vi "LVPortInitMatlab.vi"(0 "Working directory or VI Path":path, 1 "LVPort Code Lib Path (If empty auto find)":path, 5 "Code file name":string, 7 "Include path":path, 9 "Include Paths":path[](array[path]), 11 "error in":errorcluster, 12 "Autofind CodeFile if not provided":bool=TRUE) -> (4 "ID":string, 15 "error out":errorcluster)   [LabVIEW 2017]
uses:
  <userlib>/_OpenG.lib/file/file.llb/File Exists - Scalar__ogtk.vi
  <userlib>/_OpenG.lib/file/file.llb/Strip Path Extension - Path__ogtk.vi
panel:
  out "Code errors":string
  out "Create from code file":bool
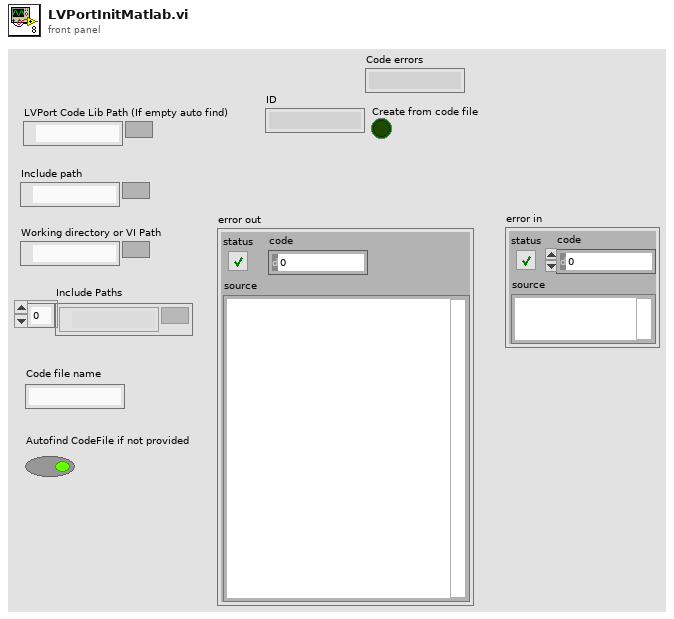
[diagram p1: front panel]
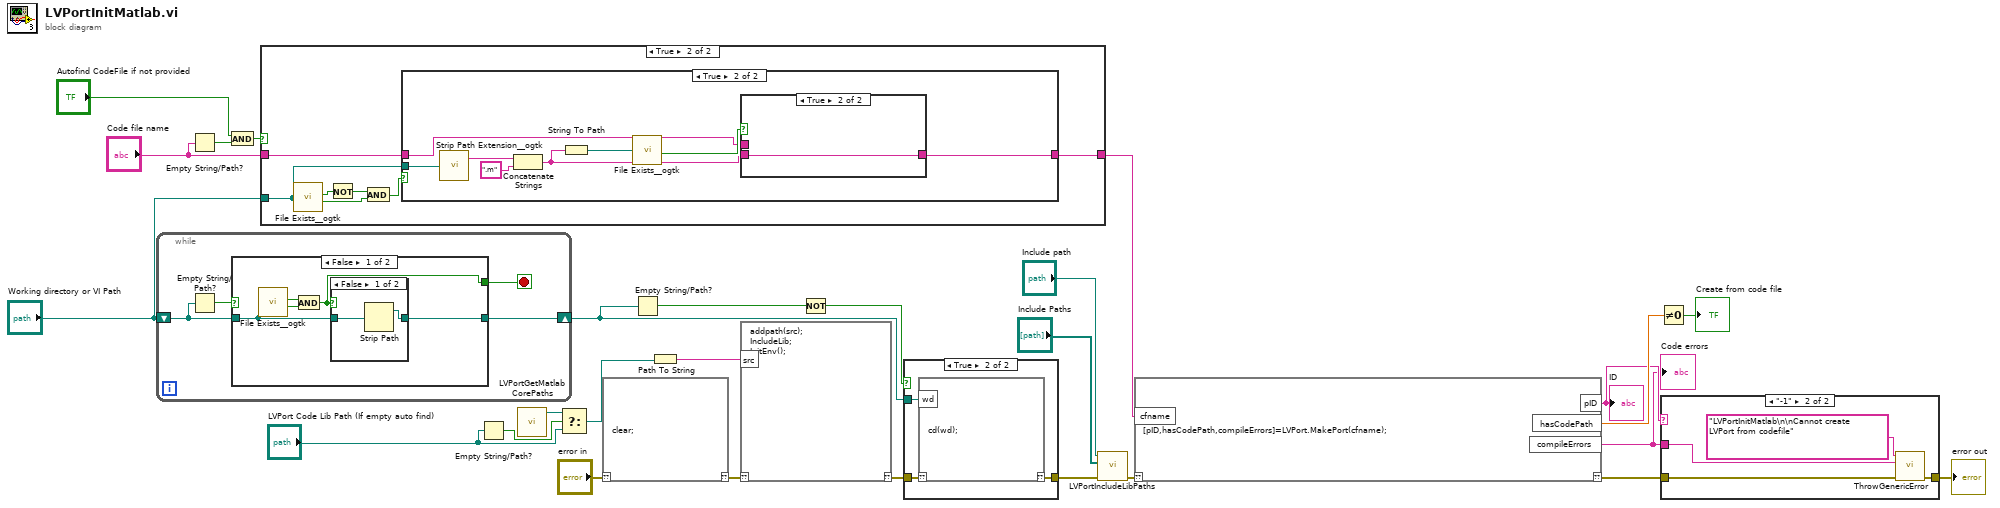
[diagram p0: block diagram]
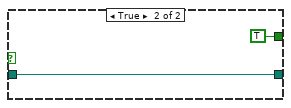
[diagram p7: hidden frame]
diagram:
  n1 = while {
    shift-right: [w30] -> w14
    shift-left: "Working directory or VI Path" -> [w31]
    stop <- w28 stop-if-true
    n2 = Empty String/Path?(string/path=w31) -> (empty?=w29:bool)
    n3 = case shown="False" w29 {
      tunnel: w31 -> [w33 w41]
      tunnel: [w36 w41] -> w30
      tunnel: [w32 TRUE ("directory")] -> w28
      frame False {
        n4 = call-poly <userlib>:"File Exists__ogtk.vi"("file path"=w33) -> ("is directory"=w35:bool, "exists"=w34:bool)  [unwired: 6 in]
        n5 = And(x=w35, y=w34) -> (x .and. y?=w32:bool)
        n6 = case shown="False" w32 {
          tunnel: w33 -> [w38 w39]
          tunnel: [w37 w39] -> w36
          frame False {
            n7 = Strip Path(path=w38) -> (stripped path=w37:path)  [unwired: 1 out]
          }
          frame True {
          }
        }
      }
      frame True {
      }
    }
  }
  n8 = Empty String/Path?(string/path="Code file name") -> (empty?=w6:bool)
  n9 = And(x="Autofind CodeFile if not provided", y=w6) -> (x .and. y?=w4:bool)
  n10 = case shown="True" w4 {
    tunnel: "Code file name" -> [w42 w45]
    tunnel: [w42 w44] -> w2
    tunnel: "Working directory or VI Path" -> [_ w43]
    frame False {
    }
    frame True {
      n11 = call-poly <userlib>:"File Exists__ogtk.vi"("file path"=w43) -> ("is directory"=w47:bool, "exists"=w46:bool)  [unwired: 6 in]
      n12 = Not(x=w47) -> (.not. x?=w48:bool)
      n13 = And(x=w48, y=w46) -> (x .and. y?=w49:bool)
      n14 = case shown="True" w49 {
        tunnel: w45 -> [w50 w57]
        tunnel: [w50 w56] -> w44
        tunnel: w43 -> [_ w52]
        frame False {
        }
        frame True {
          n15 = call-poly <userlib>:"Strip Path Extension__ogtk.vi"("path"=w52) -> ("root"=w51:string)  [unwired: 1 out]
          n16 = Concatenate Strings(w51, ".m" ("string")) -> (w53:string)
          n17 = String To Path(string=w53) -> (path=w54:path)
          n18 = call-poly <userlib>:"File Exists__ogtk.vi"("file path"=w54) -> ("exists"=w58:bool)  [unwired: 6 in, 1 out]
          n19 = case shown="True" w58 {
            tunnel: w57 -> [w59 _]
            tunnel: [w59 w60] -> w56
            tunnel: w53 -> [_ w60]
            frame False {
            }
            frame True {
            }
          }
        }
      }
    }
  }
  n20 = Empty String/Path?(string/path="LVPort Code Lib Path (If empty auto find)") -> (empty?=w26:bool)
  n21 = call "LVPortGetMatlabCorePaths.vi"() -> ("LibPath"=w20:path)  [unwired: 11 in]
  n22 = Select(t=w20, s=w26, f="LVPort Code Lib Path (If empty auto find)") -> (s? t:f=w25:path)
  n23 = script code="clear;"("??"="error in") -> ("??"=w18:errorcluster)
  n24 = Empty String/Path?(string/path=w14) -> (empty?=w24:bool)
  n25 = Path To String(path=w25) -> (string=w27:string)
  n26 = script code="addpath(src);\nIncludeLib;\nInitEnv();"("??"=w18, "src"=w27) -> ("??"=w22:errorcluster)
  n27 = Not(x=w24) -> (.not. x?=w23:bool)
  n28 = case shown="True" w23 {
    tunnel: w14 -> [_ w64]
    tunnel: w22 -> [w61 w63]
    tunnel: [w61 w62] -> w15
    frame False {
    }
    frame True {
      n29 = script code="cd(wd);"("??"=w63, "wd"=w64) -> ("??"=w62:errorcluster)
    }
  }
  n30 = call "LVPortIncludeLibPaths.vi"("error in (no error)"=w15, "Include Paths"="Include Paths", "Include path"="Include path") -> ("error out"=w13:errorcluster)  [unwired: 8 in]
  n31 = script code="[pID,hasCodePath,compileErrors]=LVPort.MakePort(cfname);"("??"=w13, "cfname"=w2) -> ("??"=w9:errorcluster, "pID"=w10:string, "hasCodePath"=w12:dbl, "compileErrors"=w8:string)
  "ID" <- w10
  "Code errors" <- w8
  n32 = Not Equal To 0?(x=w12) -> (x != 0?=→"Create from code file":bool)
  n33 = case shown="\"-1\"" w10 {
    tunnel: w9 -> [w65 w67]
    tunnel: w8 -> [_ w69]
    tunnel: [w65 w68] -> w7
    frame "False", Default {
    }
    frame "-1" {
      n34 = call "ThrowGenericError.vi"("error in (no error)"=w67, "Error info"=w69, "TheError"="LVPortInitMatlab\n\nCannot create LVPort from codefile") -> ("error out"=w68:errorcluster)  [unwired: 8 in]
    }
  }
  "error out" <- w7
